vi "writeWaitForRx.vi"(8 "error in (no error)":errorcluster, 10 "Timeout(us)":u32, 11 "ModbusBuffer in":refnum<class "ModbusBufferBuilder.lvclass">) -> (0 "error out":errorcluster, 3 "ModbusBuffer out":refnum<class "ModbusBufferBuilder.lvclass">)   [LabVIEW 2016, in "ModbusBufferBuilder.lvclass"]
uses:
  ModbusBufferBuilder.lvclass
  ModbusBufferBuilder.lvclass/ModbusBufferBuilder.ctl
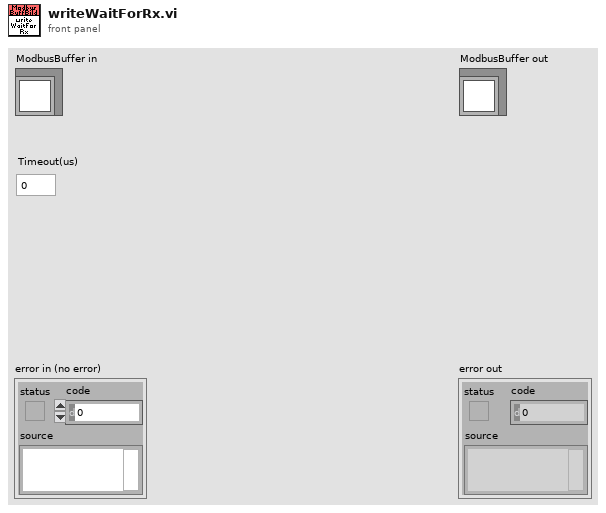
[diagram p1: front panel]
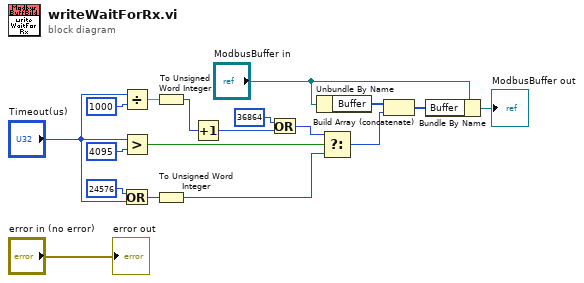
[diagram p0: block diagram]
diagram:
  n1 = Divide(x="Timeout(us)", y=u32 1000) -> (x/y=w16:dbl)
  n2 = Greater?(x="Timeout(us)", y=u32 4095) -> (0:w15:bool)
  n3 = Or(x=u16 24576, y="Timeout(us)") -> (x .or. y?=w5:u32)
  n4 = To Unsigned Word Integer(number=w16) -> (unsigned 16bit integer=w14:u16)
  n5 = To Unsigned Word Integer(number=w5) -> (unsigned 16bit integer=w4:u16)
  n6 = Increment(x=w14) -> (x+1=w9:u16)
  n7 = Or(x=u16 36864, y=w9) -> (x .or. y?=w7:u16)
  n8 = Unbundle By Name("ModbusBuffer in") -> ("Buffer"=w2:u16[])
  n9 = Select(t=w7, s=w15, f=w4) -> (s? t:f=w3:u16)
  n10 = Build Array (concatenate)(w2, w3) -> (w1:u16[])
  n11 = Bundle By Name(cluster="ModbusBuffer in", "Buffer"=w1) -> (→"ModbusBuffer out":refnum<class "ModbusBufferBuilder.lvclass">)
  "error out" <- "error in (no error)"
